vi "setObjectPrivateData.vi"(7 "error in (no error)":errorcluster, 9 "privateData":variant[](array[variant]), 10 "object in":refnum<class>) -> (0 "error out":errorcluster, 3 "object out":refnum<class>)   [LabVIEW 2020, in "JKI JSON Object Serialization.lvlib" / "OOP_Utility.lvlib" / "Reflection.lvclass"]
doc: "Applies 'privateData' to the input object where privateData is an array of Variants where each element is the cluster of private data for a class in the hierarchy. \n\nGCraftsman JSON Object Serialization Toolkit\nwww.GCraftsman.com\nCopyright (c) 2017, GCraftsman"
uses:
  Reflection.lvclass
  reflectionPool.vi
  Reflection.lvclass/Reflection.ctl
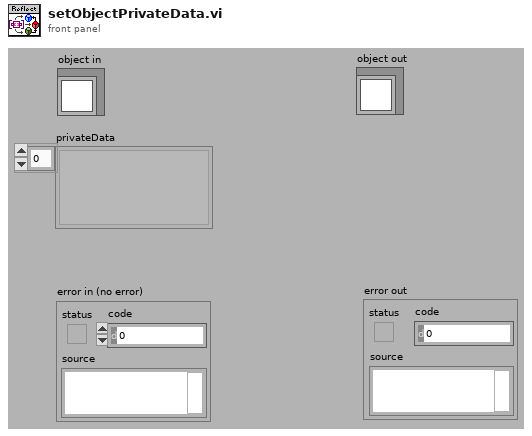
[diagram p1: front panel]
types:
  T1 = cluster{"Major":u16, "Minor":u16, "Fix":u16, "Build":u16}[]
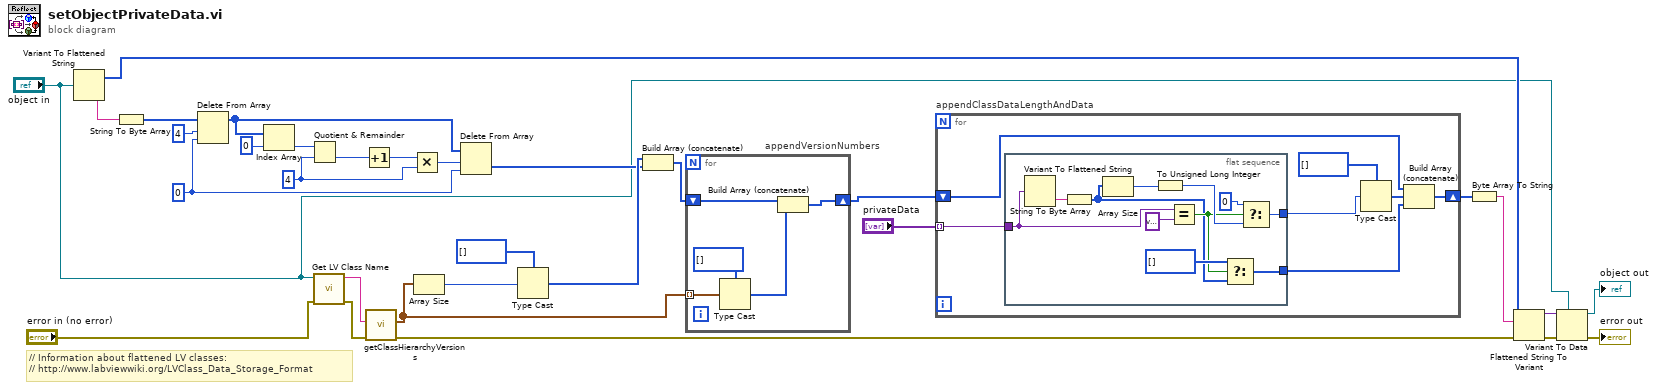
[diagram p0: block diagram]
diagram:
  w22 = u8 4 ("y")
  w29 = 0 ("index")
  # "// Information about flattened LV classes:\n// http://www.labviewwiki.org/LVClass_Data_Storage_Format"
  n1 = Variant To Flattened String(Variant="object in") -> (data string=w31:string, 1:w21:i16[])
  n2 = String To Byte Array(string=w31) -> (unsigned byte array=w28:u8[])
  n3 = Delete From Array(array=w28, length=4 ("offset (0)"), index=w29) -> (array with subset deleted=w30:u8[])  [unwired: 1 out]
  n4 = Index Array(array=w30, index=0) -> (element=w25:u8)
  n5 = Quotient & Remainder(x=w25, y=w22) -> (floor(x/y)=w24:u8)  [unwired: 1 out]
  n6 = call <vilib>:"Get LV Class Name.vi"("error in (no error)"="error in (no error)", "object"="object in") -> ("error out"=w1:errorcluster, "class name"=w6:string)  [unwired: 8 in]
  n7 = Increment(x=w24) -> (x+1=w23:u8)
  n8 = call "getClassHierarchyVersions.vi"("error in"=w1, "className"=w6) -> ("error out"=w8:errorcluster, "allClassVersionNumbers"=w3:T1)  [unwired: 8 in]
  n9 = Multiply(x=w23, y=w22) -> (x*y=w20:u8)
  n10 = Array Size(array=w3) -> (size(s)=w2:i32)
  n11 = Delete From Array(array=w30, length=w20, index=w29) -> (deleted portion=w14:u8[])  [unwired: 1 out]
  n12 = Type Cast(type=u8[] [] ("unsigned byte array"), x=w2) -> (*(type *) &x=w15:u8[])
  n13 = Build Array (concatenate)(w15, w14) -> (w11:u8[])
  n14 = for "appendVersionNumbers" {
    shift-right: [w36] -> w10
    shift-left: w11 -> [w33]
    tunnel: w3 -> [w35] mode=indexing
    n15 = Type Cast(type=u8[] [] ("unsigned byte array"), x=w35) -> (*(type *) &x=w34:u8[])
    n16 = Build Array (concatenate)(w33, w34) -> (w36:u8[])
  }
  n17 = for "appendClassDataLengthAndData" {
    shift-right: [w42] -> w13
    shift-left: w10 -> [w43]
    tunnel: "privateData" -> [w37] mode=indexing
    n18 = flat-sequence {
      tunnel: [w46] -> w39
      tunnel: [w45] -> w38
      tunnel: w37 -> [w44]
      frame #0 {
        n19 = Variant To Flattened String(Variant=w44) -> (data string=w47:string)  [unwired: 1 out]
        n20 = String To Byte Array(string=w47) -> (unsigned byte array=w49:u8[])
        n21 = Array Size(array=w49) -> (size(s)=w52:i32)
        n22 = To Unsigned Long Integer(number=w52) -> (unsigned 32bit integer=w53:u32)
        n23 = Equal?(x=w44, y=variant ("element")) -> (x = y?=w50:bool)
        n24 = Select(t=u8[] [], s=w50, f=w49) -> (s? t:f=w45:u8[])
        n25 = Select(t=u32 0, s=w50, f=w53) -> (s? t:f=w46:u32)
      }
    }
    n26 = Type Cast(type=u8[] [] ("unsigned byte array"), x=w39) -> (*(type *) &x=w40:u8[])
    n27 = Build Array (concatenate)(w43, w40, w38) -> (w42:u8[])
  }
  n28 = Byte Array To String(unsigned byte array=w13) -> (string=w12:string)
  n29 = Flattened String To Variant(4:w8, 6:w12, 7:w21) -> (0:w9:errorcluster, 3:w17:variant)
  n30 = Variant To Data(error in=w9, type="object in", Variant=w17) -> (data=→"object out":refnum<class>, error out=→"error out":errorcluster)
